vi "PID Change Detect.vi"(8 "FF":dbl, 9 "D":dbl, 10 "I":dbl, 11 "P":dbl) -> (2 "Changed?":bool)   [LabVIEW 2016]
uses:
  Common Code/Utilities/Change Detect Double.vi
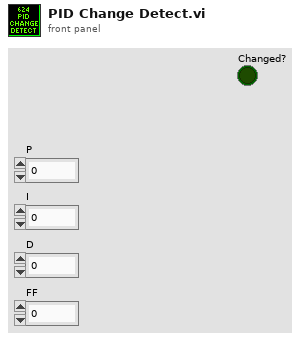
[diagram p1: front panel]
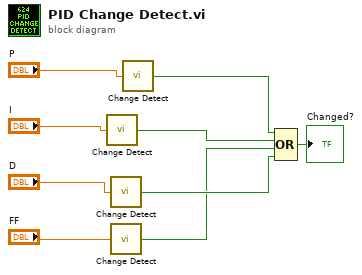
[diagram p0: block diagram]
diagram:
  n1 = call-poly "Change Detect.vi"("In"="I") -> ("Changed?"=w4:bool)
  n2 = call-poly "Change Detect.vi"("In"="D") -> ("Changed?"=w3:bool)
  n3 = call-poly "Change Detect.vi"("In"="FF") -> ("Changed?"=w2:bool)
  n4 = call-poly "Change Detect.vi"("In"="P") -> ("Changed?"=w5:bool)
  n5 = Compound Arithmetic op=OR(w5, w4, w2, w3) -> (→"Changed?":bool)
